vi "Live Z Scale Update.vi"(0 "IMAQ Display Refs":refnum<vi>[](array[refnum]), 11 "Z Scale Refs":refnum<vi>[](array[refnum])) -> ()   [LabVIEW 2016]
uses:
  <vilib>/vision/Image Controls.llb/IMAQ Image.ctl
  <vilib>/vision/NI_Vision_Development_Module.lvlib
panel:
  out "Error":errorcluster
  # "Copyright (C) 2020 Edward S Allgeyer\n\nRedistribution and use in source and binary forms, with or without\nmodification, are permitted provided that the following conditions\nare met:\n\n1. Redistributions of source code must retain the above copyright\n   notice, this list of conditions and the following disclaimer.\n\n2. Redistributions in binary form must reproduce the above copyright\n   notice, this list of conditions and the following disclaimer in\n   the documentation and/or other materials provided with the\n   distribution.\n\n3. Neither the name of the copyright holder nor the names of its\n   contributors may be used to endorse or promote products derived\n   from this software without specific prior written permission.\n\nTHIS SOFTWARE IS PROVIDED BY THE COPYRIGHT HOLDERS AND CONTRIBUTORS\n\"AS IS\" AND ANY EXPRESS OR IMPLIED WARRANTIES, INCLUDING, BUT NOT\nLIMITED TO, THE IMPLIED WARRANTIES OF MERCHANTABILITY AND FITNESS\nFOR A PARTICULAR PURPOSE ARE DISCLAIMED. IN NO EVENT SHALL THE\nCOPYRIGHT HOLDER OR CONTRIBUTORS BE LIABLE FOR ANY DIRECT, INDIRECT,\nINCIDENTAL, SPECIAL, EXEMPLARY, OR CONSEQUENTIAL DAMAGES (INCLUDING,\nBUT NOT LIMITED TO, PROCUREMENT OF SUBSTITUTE GOODS OR SERVICES;\nLOSS OF USE, DATA, OR PROFITS; OR BUSINESS INTERRUPTION) HOWEVER\nCAUSED AND ON ANY THEORY OF LIABILITY, WHETHER IN CONTRACT, STRICT\nLIABILITY, OR TORT (INCLUDING NEGLIGENCE OR OTHERWISE) ARISING IN\nANY WAY OUT OF THE USE OF THIS SOFTWARE, EVEN IF ADVISED OF THE\nPOSSIBILITY OF SUCH DAMAGE."
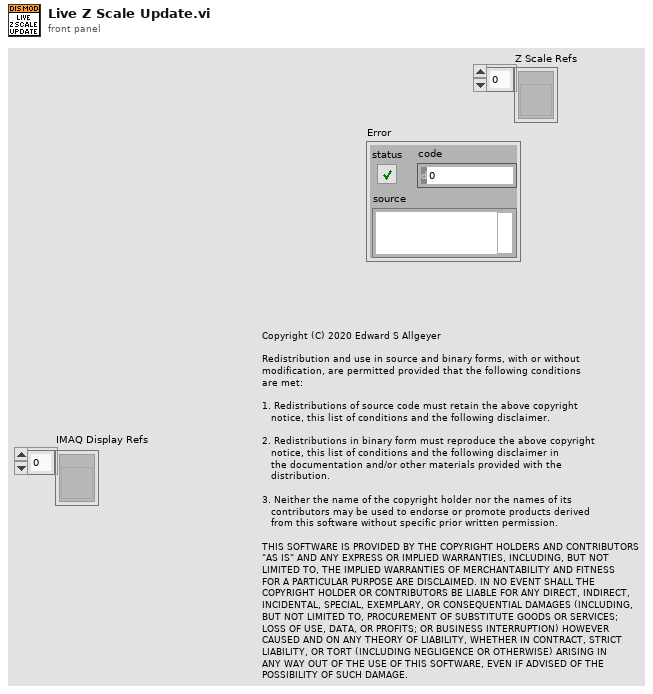
[diagram p1: front panel]
types:
  T1 = typedef "IMAQ Image.ctl" = refnum<image>
  T2 = cluster{"Mean Value":sgl, "Standard Variation":sgl, "Minimal Value":sgl, "Maximal Value":sgl, "Area (calibrated)":sgl, "Area (pixels)":u32, "%":sgl, "Calibration Valid":bool}
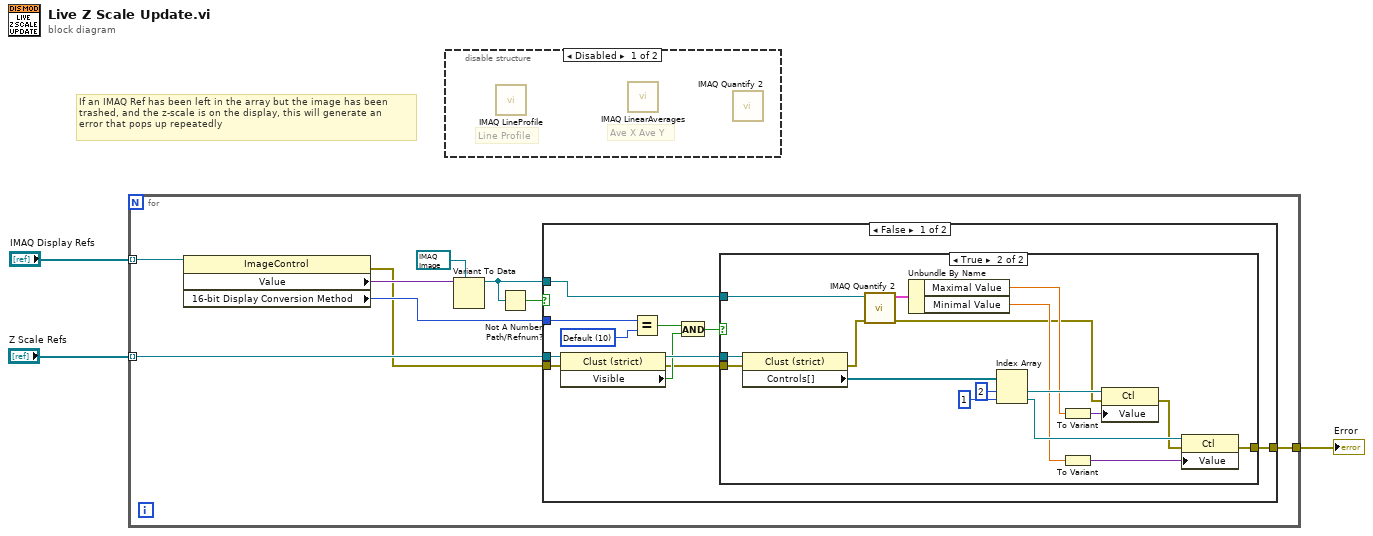
[diagram p0: block diagram]
diagram:
  # "If an IMAQ Ref has been left in the array but the image has been\ntrashed, and the z-scale is on the display, this will generate an\nerror that pops up repeatedly"
  n1 = for {
    tunnel: "IMAQ Display Refs" -> [w12] mode=indexing
    tunnel: "Z Scale Refs" -> [w6] mode=indexing
    tunnel: [w4] -> w1
    n2 = property class="ImageControl"(reference=w12) -> (error out=w5:errorcluster, "Value"=w11:variant, "16-bit Display Conversion Method"=w7:u32)  [unwired: 1 in, 1 out]
    n3 = Variant To Data(type=T1 refnum ("New Image"), Variant=w11) -> (data=w9:T1)  [unwired: 1 in, 1 out]
    n4 = Not A Number/Path/Refnum?(number/path/refnum=w9) -> (NaN/Path/Refnum?=w8:bool)
    n5 = case shown="False" w8 {
      tunnel: w9 -> [w21 _]
      tunnel: w6 -> [w20 _]
      tunnel: w7 -> [w23 _]
      tunnel: w5 -> [w15 w42]
      tunnel: [w13 w42] -> w4
      frame False {
        w22 = u32 10 items=["Default"=10, "Most Significant Bits"=11, "Full Dynamic"=12, "Downshift"=13, "Given Range"=14, "90% Dynamic"=15, "Given Percent Range"=16] ("16-bit Display Mapping:Conversion Method")
        n6 = property class="Clust (strict)"(reference=w20, error in=w15) -> (reference out=w19:refnum<vi>, error out=w14:errorcluster, "Visible"=w17:bool)
        n7 = Equal?(x=w23, y=w22) -> (x = y?=w18:bool)
        n8 = And(x=w18, y=w17) -> (x .and. y?=w16:bool)
        n9 = case shown="True" w16 {
          tunnel: w19 -> [_ w41]
          tunnel: w21 -> [_ w33]
          tunnel: w14 -> [w24 w29]
          tunnel: [w24 w25] -> w13
          frame False {
          }
          frame True {
            n10 = property class="Clust (strict)"(reference=w41, error in=w29) -> (error out=w28:errorcluster, "Controls[]"=w40:refnum<vi>[])  [unwired: 1 out]
            n11 = call "IMAQ Quantify 2"("error in (no error)"=w28, "Image"=w33) -> ("error out"=w27:errorcluster, "Global Report"=w32:T2)  [unwired: 7 in, 1 out]
            n12 = Unbundle By Name(w32) -> ("Maximal Value"=w30:sgl, "Minimal Value"=w31:sgl)
            n13 = Index Array(array=w40, index #1=2 ("index"), index #2=1 ("index")) -> (element #1=w37:refnum<vi>, element #2=w36:refnum<vi>)
            n14 = To Variant(anything=w30) -> (Variant=w35:variant)
            n15 = To Variant(anything=w31) -> (Variant=w34:variant)
            n16 = property class="Ctl"(reference=w37, error in=w27, "Value"=w35) -> (error out=w26:errorcluster)  [unwired: 1 out]
            n17 = property class="Ctl"(reference=w36, error in=w26, "Value"=w34) -> (error out=w25:errorcluster)  [unwired: 1 out]
          }
        }
      }
      frame True {
      }
    }
  }
  "Error" <- w1
  n18 = disable-structure shown="Disabled" {
    frame Disabled {
      # "Ave X Ave Y"
      # "Line Profile"
      n19 = call "IMAQ LineProfile"() -> ()  [unwired: 5 in, 4 out]
      n20 = call "IMAQ LinearAverages"() -> ()  [unwired: 7 in, 5 out]
      n21 = call "IMAQ Quantify 2"() -> ()  [unwired: 9 in, 3 out]
    }
    frame Enabled {
    }
  }
